vi "MoveWin.vi"(6 "SecondsToRetry":i32=2, 8 "error in (no error)":errorcluster, 9 "Window Name":string, 10 "Left":i16, 11 "Top":i16) -> (0 "error out":errorcluster)   [LabVIEW 2020, in "WinAPI.lvlib"]
uses:
  WinAPI.lvlib
  C:/Users/dzoni/Documents/NJ/Playground/LV/WinAPI/DLL/WinAPI.dll
  DLL/WinAPI.dll
  System.Drawing
  1181b3a2-8b9c-4c58-917e-629617c933e7.vi
panel:
  out "iter":i32
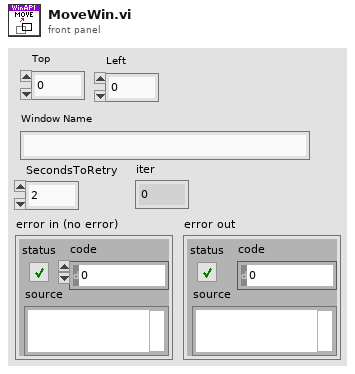
[diagram p1: front panel]
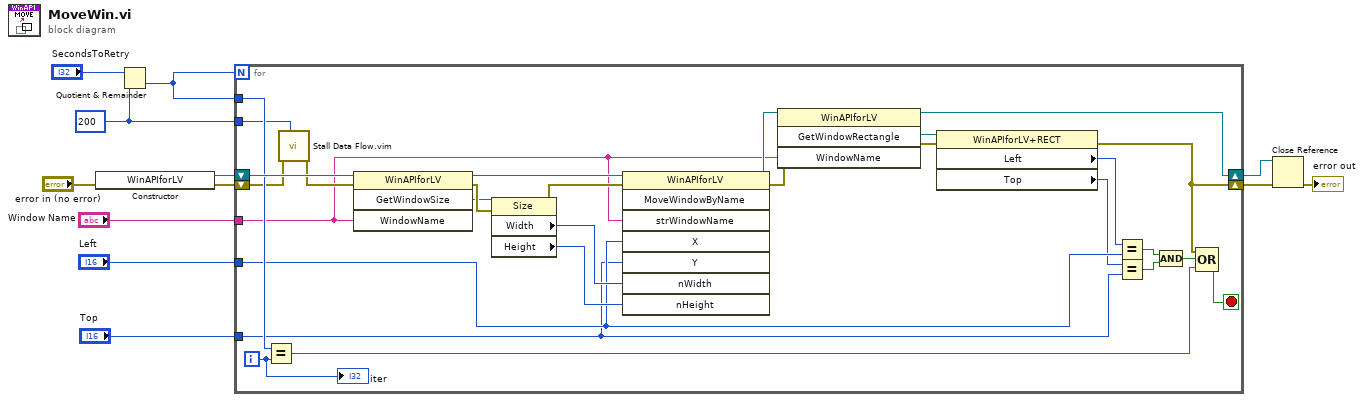
[diagram p0: block diagram]
diagram:
  w2 = u32 200 ("milliseconds to wait")
  n1 = constructor class="WinAPIforLV"(error in="error in (no error)") -> (reference out=w6:refnum<k24>, error out=w8:errorcluster)  [unwired: 2 in, 1 out]
  n2 = Quotient & Remainder(x="SecondsToRetry", y=w2) -> (floor(x/y)=w1:u32)  [unwired: 1 out]
  n3 = for {
    N: w1 -> [_]
    tunnel: "Top" -> [w14]
    tunnel: "Left" -> [w19]
    tunnel: "Window Name" -> [w13]
    shift-right: [w21] -> w9
    shift-left: w8 -> [w29]
    shift-right: [w23] -> w7
    shift-left: w6 -> [w40]
    tunnel: w1 -> [w31]
    tunnel: w2 -> [w27]
    i -> [w32]
    stop <- w33 stop-if-true
    n4 = Equal?(x=w31, y=w32) -> (x = y?=w30:bool)
    n5 = call "Stall Data Flow.vim"("value in"=w29, "milliseconds to wait"=w27) -> ("value out"=w28:errorcluster)  [unwired: 1 out]
    n6 = invoke class="WinAPIforLV" method="GetWindowSize"(reference=w40, error in=w28, "WindowName"=w13) -> (reference out=w37:refnum<k24>, error out=w38:errorcluster, "GetWindowSize"=w34:refnum<k24>)  [unwired: 1 in, 1 out]
    n7 = property class="Size"(reference=w34, error in=w38) -> (error out=w39:errorcluster, "Width"=w35:i32, "Height"=w36:i32)  [unwired: 1 out]
    n8 = invoke class="WinAPIforLV" method="MoveWindowByName"(reference=w37, error in=w39, "strWindowName"=w13, "X"=w19, "Y"=w14, "nWidth"=w35, "nHeight"=w36) -> (reference out=w24:refnum<k24>, error out=w25:errorcluster)  [unwired: 1 in, 6 out]
    n9 = invoke class="WinAPIforLV" method="GetWindowRectangle"(reference=w24, error in=w25, "WindowName"=w13) -> (reference out=w23:refnum<k24>, error out=w22:errorcluster, "GetWindowRectangle"=w26:refnum<k24>)  [unwired: 1 in, 1 out]
    n10 = property class="WinAPIforLV+RECT"(reference=w26, error in=w22) -> (error out=w21:errorcluster, "Left"=w20:i32, "Top"=w15:i32)  [unwired: 1 out]
    n11 = Equal?(x=w20, y=w19) -> (x = y?=w17:bool)
    n12 = Equal?(x=w15, y=w14) -> (x = y?=w18:bool)
    n13 = Compound Arithmetic op=AND(w17, w18) -> (w16:bool)
    n14 = Compound Arithmetic op=OR(w21, w16, w30) -> (w33:bool)
    "iter" <- w32
  }
  n15 = Close Reference(reference=w7, error in (no error)=w9) -> (error out=→"error out":errorcluster)
